vi "Get Next Available Slot.vi"(8 "error in (no error)":errorcluster, 11 "Device Ref in":T1 format="%.0x") -> (0 "error out":errorcluster, 2 "Next Open Slot":T2 {"Slot #" max=15}, 3 "Device Ref out":T1 format="%.0x")   [LabVIEW 2014, in "SLSC configuration System Explorer.lvlib"]
uses:
  SLSC configuration System Explorer.lvlib
  <vilib>/NI Veristand/Custom Device API/Custom Device Item Ref.ctl
  Type Defs/Card Position.ctl
  Shared/SPI Utility/Slot #.ctl
  Shared/Constants.vi
  <vilib>/NI Veristand/Custom Device API/Get Item Property (U32).vi
  <vilib>/NI Veristand/Custom Device API/Custom Device API.lvlib
  Shared/SLSC configuration Shared.lvlib
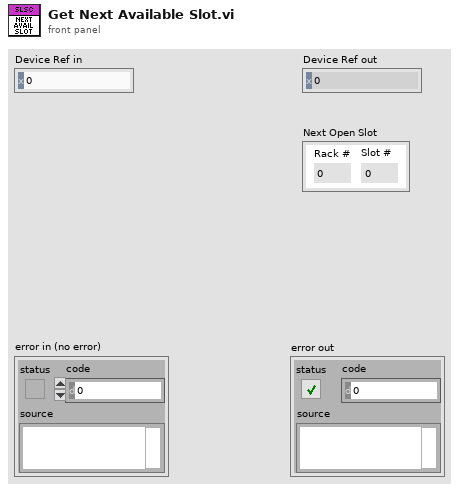
[diagram p1: front panel]
types:
  T1 = typedef "Custom Device API.lvlib/Custom Device Item Ref.ctl" = u64
  T2 = typedef "SLSC configuration Shared.lvlib/Card Position.ctl" = cluster{"Rack #":u8, "Slot #":T3}
  T3 = typedef "SLSC configuration Shared.lvlib/Slot #.ctl" = u8
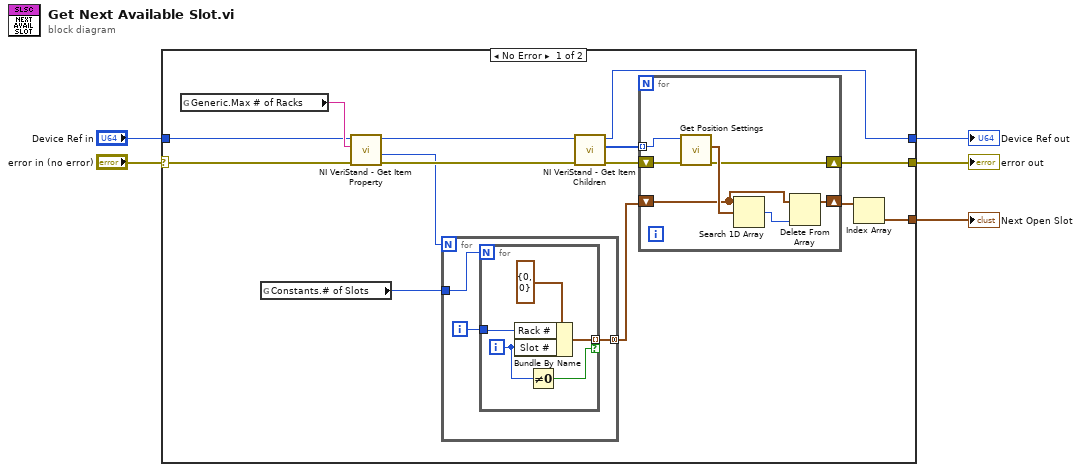
[diagram p0: block diagram]
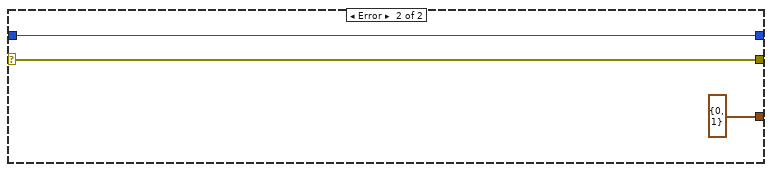
[diagram p2: hidden frame]
diagram:
  n1 = case shown="No Error" "error in (no error)" {
    selector: "error in (no error)" -> [w13 w36]
    tunnel: "Device Ref in" -> [w14 w37]
    tunnel: [w18 T2 {"Rack #"=0, "Slot #"=1} ("Card Position")] -> w4
    tunnel: [w17 w36] -> w3
    tunnel: [w16 w37] -> w2
    frame No Error {
      n2 = global read "Constants.vi" "Generic.Max # of Racks"() -> (w15:string)
      n3 = global read "Constants.vi" "Constants.# of Slots"() -> (w19:u8)
      n4 = call-poly <vilib>:"NI VeriStand - Get Item Property.vi"("error in (no error)"=w13, "Property Name"=w15, "Item Ref in"=w14) -> ("error out"=w12:errorcluster, "Value"=w10:u32, "Item Ref out"=w11:T1)  [unwired: 5 in, 1 out]
      n5 = for {
        N: w10 -> [_]
        tunnel: w19 -> [w29]
        tunnel: [w27] -> w8 mode=concatenating
        i -> [w28]
        n6 = for {
          N: w29 -> [_]
          tunnel: w28 -> [w34]
          tunnel: [w32] -> w27 mode=indexing if=w30
          i -> [w31]
          n7 = Bundle By Name(cluster=T2 {"Rack #"=0, "Slot #"=0} ("Card Position"), "Rack #"=w34, "Slot #"=w31) -> (w32:T2)
          n8 = Not Equal To 0?(x=w31) -> (x != 0?=w30:bool)
        }
      }
      n9 = call <vilib>:"NI VeriStand - Get Item Children.vi"("error in (no error)"=w12, "Item Ref in"=w11) -> ("error out"=w7:errorcluster, "Child Refs"=w9:T1[], "Item Ref out"=w16:T1)  [unwired: 6 in, 1 out]
      n10 = for {
        tunnel: w9 -> [w26] mode=indexing
        shift-right: [w20] -> w6
        shift-left: w8 -> [w21]
        shift-right: [w23] -> w17
        shift-left: w7 -> [w25]
        n11 = call "Get Position Settings.vi"("error in (no error)"=w25, "Item Ref in"=w26) -> ("error out"=w23:errorcluster, "Card Position"=w24:T2)  [unwired: 7 in, 1 out]
        n12 = Search 1D Array(1D array=w21, element=w24) -> (index of element=w22:i32)  [unwired: 1 in]
        n13 = Delete From Array(array=w21, index=w22) -> (array with subset deleted=w20:T2[])  [unwired: 1 in, 1 out]
      }
      n14 = Index Array(array=w6) -> (element=w18:T2)  [unwired: 1 in]
    }
    frame Error {
    }
  }
  "Next Open Slot" <- w4
  "error out" <- w3
  "Device Ref out" <- w2
